vi "Add When VIs.vi"(8 "error in (no error)":errorcluster, 11 "Mock Class Generator In":refnum<class "Mock Class Generator.lvclass">) -> (0 "error out":errorcluster, 2 "When VIs":path[](array[path]), 3 "Mock Class Generator Out":refnum<class "Mock Class Generator.lvclass">)   [LabVIEW 2020, in "Mock Class Generator.lvclass"]
uses:
  Mock Class Generator.lvclass
  Mock Class Generator.lvclass/Mock Class Generator.ctl
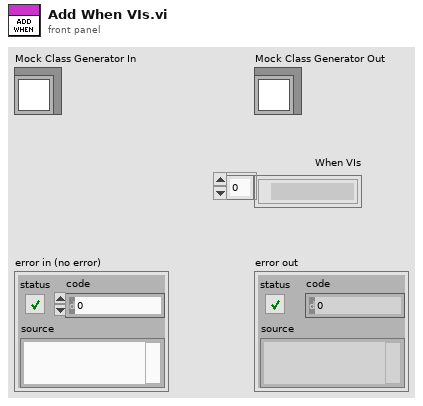
[diagram p1: front panel]
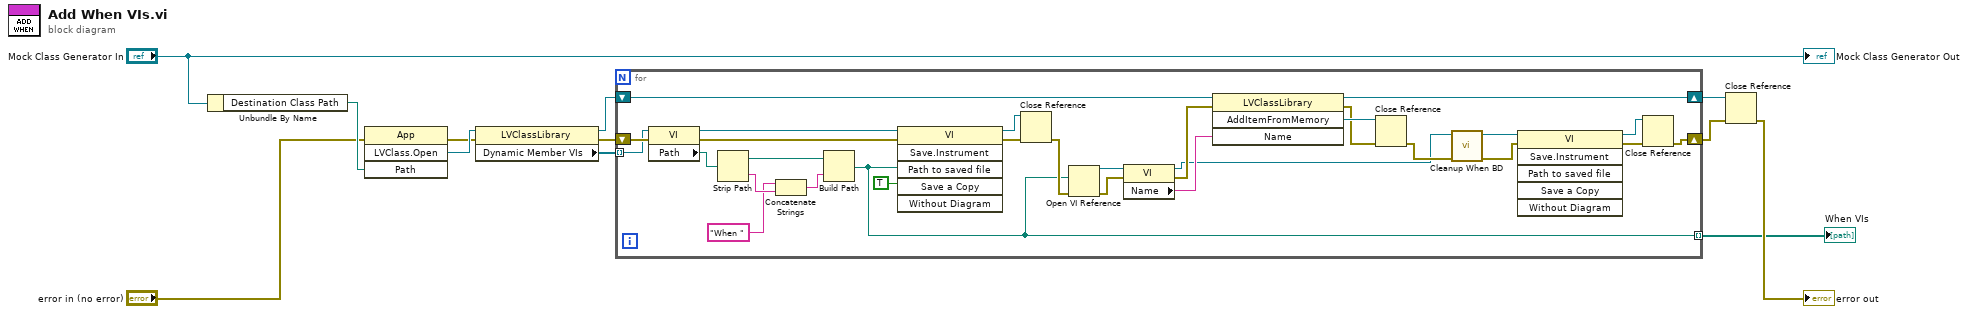
[diagram p0: block diagram]
diagram:
  n1 = Unbundle By Name("Mock Class Generator In") -> ("Destination Class Path"=w8:path)
  n2 = invoke class="App" method="LVClass.Open"(error in="error in (no error)", "Path"=w8) -> (error out=w11:errorcluster, "LVClass.Open"=w12:refnum<vi>)  [unwired: 2 in, 2 out]
  n3 = property class="LVClassLibrary"(reference=w12, error in=w11) -> (reference out=w6:refnum<vi>, error out=w10:errorcluster, "Dynamic Member VIs"=w7:refnum<vi>[])
  n4 = for {
    tunnel: w7 -> [w34] mode=indexing
    shift-right: [w16] -> w4
    shift-left: w10 -> [w35]
    shift-right: [w23] -> w5
    shift-left: w6 -> [w27]
    tunnel: [w15] -> w1 mode=indexing
    n5 = property class="VI"(reference=w34, error in=w35) -> (reference out=w39:refnum<vi>, error out=w38:errorcluster, "Path"=w41:path)
    n6 = Strip Path(path=w41) -> (stripped path=w33:path, name=w32:string)
    n7 = Concatenate Strings("When " ("string"), w32) -> (w30:string)
    n8 = Build Path(base path=w33, name or relative path=w30) -> (appended path=w15:path)
    n9 = invoke class="VI" method="Save.Instrument"(reference=w39, error in=w38, "Path to saved file"=w15, "Save a Copy"=TRUE) -> (reference out=w36:refnum<vi>, error out=w37:errorcluster)  [unwired: 2 in, 4 out]
    n10 = Close Reference(reference=w36, error in (no error)=w37) -> (error out=w26:errorcluster)
    n11 = Open VI Reference(vi path=w15, error in (no error)=w26) -> (vi reference=w25:refnum<vi>, error out=w24:errorcluster)  [unwired: 4 in]
    n12 = property class="VI"(reference=w25, error in=w24) -> (reference out=w17:refnum<vi>, error out=w28:errorcluster, "Name"=w29:string)
    n13 = invoke class="LVClassLibrary" method="AddItemFromMemory"(reference=w27, error in=w28, "Name"=w29) -> (reference out=w23:refnum<vi>, error out=w19:errorcluster, "AddItemFromMemory"=w20:refnum<vi>)  [unwired: 1 in, 1 out]
    n14 = Close Reference(reference=w20, error in (no error)=w19) -> (error out=w18:errorcluster)
    n15 = call "Cleanup When BD.vi"("error in (no error)"=w18, "VI in"=w17) -> ("error out"=w14:errorcluster, "VI out"=w13:refnum<vi>)  [unwired: 8 in]
    n16 = invoke class="VI" method="Save.Instrument"(reference=w13, error in=w14) -> (reference out=w22:refnum<vi>, error out=w21:errorcluster)  [unwired: 4 in, 4 out]
    n17 = Close Reference(reference=w22, error in (no error)=w21) -> (error out=w16:errorcluster)
  }
  "When VIs" <- w1
  n18 = Close Reference(reference=w5, error in (no error)=w4) -> (error out=→"error out":errorcluster)
  "Mock Class Generator Out" <- "Mock Class Generator In"
